vi "new gimbal.vi"(8 "error in \n(no error)":errorcluster) -> (0 "error out":errorcluster, 3 "Data":T1)   [LabVIEW 2015]
uses:
  typedefs/gimbal data.ctl
  <vilib>/picture/3D Picture Control/NI_3D Picture Control.lvlib
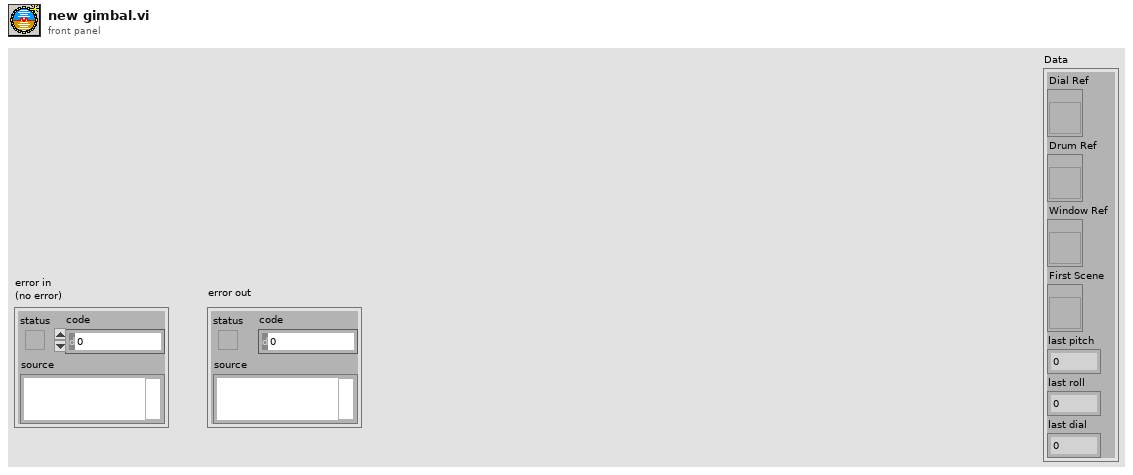
[diagram p1: front panel]
types:
  T1 = typedef "gimbal data.ctl" = cluster{"Dial Ref":refnum<vi>, "Drum Ref":refnum<vi>, "Window Ref":refnum<vi>, "First Scene":refnum<vi>, "last pitch":dbl, "last roll":dbl, "last dial":dbl}
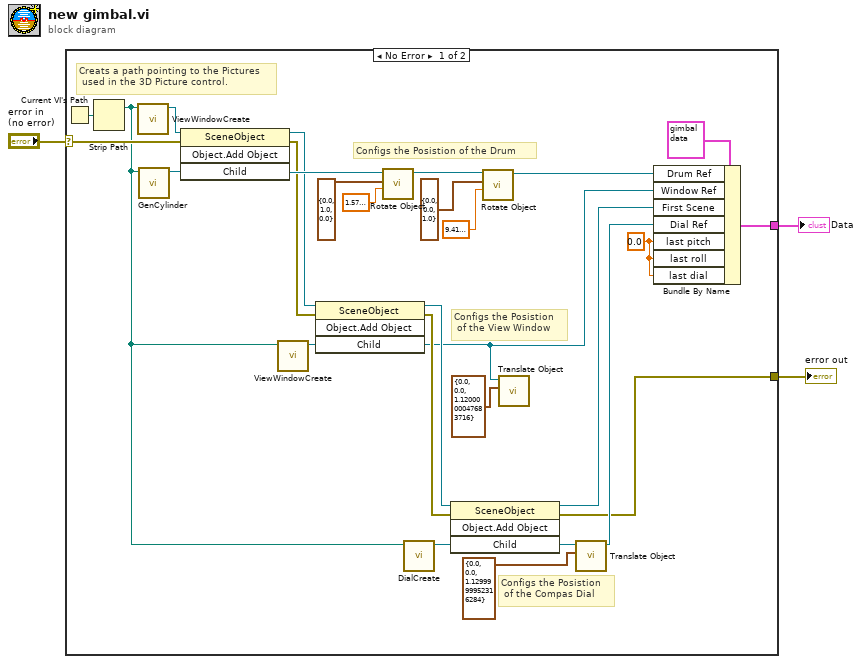
[diagram p0: block diagram]
diagram:
  n1 = case shown="No Error" "error in \n(no error)" {
    selector: "error in \n(no error)" -> [w18 w32]
    tunnel: [w6 w32] -> w2
    tunnel: [w5 _] -> w1
    frame No Error {
      w4 = 0.0 ("last pitch")
      # "Configs the Posistion\n of the Compas Dial"
      # "Configs the Posistion\n of the View Window"
      # "Configs the Posistion of the Drum"
      # "Creats a path pointing to the Pictures\n used in the 3D Picture control."
      n2 = Current VI's Path() -> (path=w15:path)
      n3 = Strip Path(path=w15) -> (stripped path=w13:path)  [unwired: 1 out]
      n4 = call "ViewWindowCreate.vi"("Solid Horizon Path.PNG"=w13) -> ("SceneObject out"=w14:refnum<vi>)  [unwired: 10 in]
      n5 = call "GenCylinder.vi"("Solid Horizon Path.PNG"=w13) -> ("SceneObject out"=w29:refnum<vi>)  [unwired: 10 in]
      n6 = invoke class="SceneObject" method="Object.Add Object"(reference=w14, error in=w18, "Child"=w29) -> (reference out=w19:refnum<vi>, error out=w17:errorcluster, "Child"=w23:refnum<vi>)  [unwired: 1 in, 1 out]
      n7 = call "ViewWindowCreate.vi"("Solid Horizon Path.PNG"=w13) -> ("SceneObject out"=w12:refnum<vi>)  [unwired: 10 in]
      n8 = invoke class="SceneObject" method="Object.Add Object"(reference=w19, error in=w17, "Child"=w12) -> (reference out=w31:refnum<vi>, error out=w16:errorcluster, "Child"=w9:refnum<vi>)  [unwired: 1 in, 1 out]
      n9 = call <vilib>:"Rotate Object.vi"("Angle"=sgl 1.5799999 ("Angle 2"), "Axis"=cluster{"X":sgl, "Y":sgl, "Z":sgl} {"X"=0.0, "Y"=1.0, "Z"=0.0} ("Axis 2"), "Scene.Object In"=w23) -> ("Scene.Object Out"=w22:refnum<vi>)  [unwired: 7 in, 1 out]
      n10 = call "DialCreate.vi"("Solid Horizon Path.PNG"=w13) -> ("SceneObject out"=w30:refnum<vi>)  [unwired: 10 in]
      n11 = invoke class="SceneObject" method="Object.Add Object"(reference=w31, error in=w16, "Child"=w30) -> (reference out=w8:refnum<vi>, error out=w6:errorcluster, "Child"=w26:refnum<vi>)  [unwired: 1 in, 1 out]
      n12 = call <vilib>:"Rotate Object.vi"("Angle"=sgl 9.419999 ("Angle 3"), "Axis"=cluster{"X":sgl, "Y":sgl, "Z":sgl} {"X"=0.0, "Y"=0.0, "Z"=1.0} ("Axis 3"), "Scene.Object In"=w22) -> ("Scene.Object Out"=w10:refnum<vi>)  [unwired: 7 in, 1 out]
      n13 = call <vilib>:"Translate Object.vi"("Translation"=cluster{"X":sgl, "Y":sgl, "Z":sgl} {"X"=0.0, "Y"=0.0, "Z"=1.12} ("Translation 4"), "Scene.Object In"=w9) -> ()  [unwired: 8 in, 2 out]
      n14 = call <vilib>:"Translate Object.vi"("Translation"=cluster{"X":sgl, "Y":sgl, "Z":sgl} {"X"=0.0, "Y"=0.0, "Z"=1.13} ("Translation 5"), "Scene.Object In"=w26) -> ("Scene.Object Out"=w7:refnum<vi>)  [unwired: 8 in, 1 out]
      n15 = Bundle By Name(cluster=T1 {"Dial Ref"=refnum, "Drum Ref"=refnum, "Window Ref"=refnum, "First Scene"=refnum, "last pitch"=0.0, "last roll"=0.0, "last dial"=0.0}, "Drum Ref"=w10, "Window Ref"=w9, "First Scene"=w8, "Dial Ref"=w7, "last pitch"=w4, "last roll"=w4, "last dial"=w4) -> (w5:T1)
    }
    frame Error {
    }
  }
  "error out" <- w2
  "Data" <- w1
